vi "Test 3.vi"() -> ()   [LabVIEW 2016, in "Drona basic.lvlib"]
uses:
  Drona basic.lvlib
  Test 2.vi
panel:
  in  "Tab Control":enum32{"Page 1", "Page 2"}(tab)
  in  "Numeric 3":i32=100
  in  "Boolean":bool
  in  "Numeric 2":dbl
  in  "Numeric":dbl
  in  "error in (no error)":errorcluster
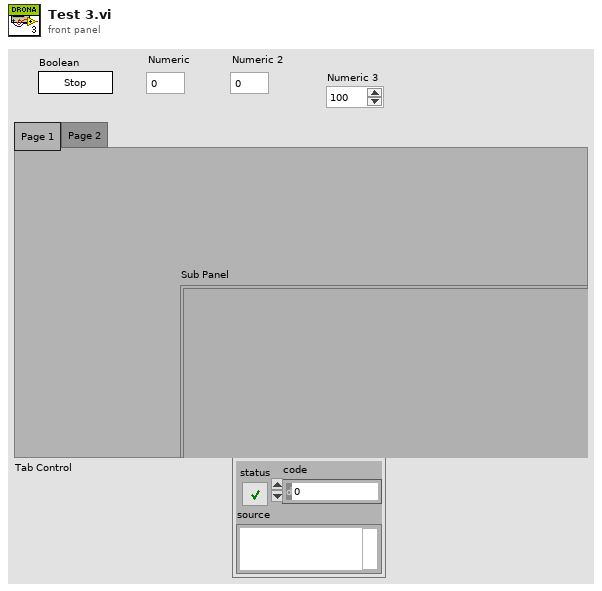
[diagram p1: front panel]
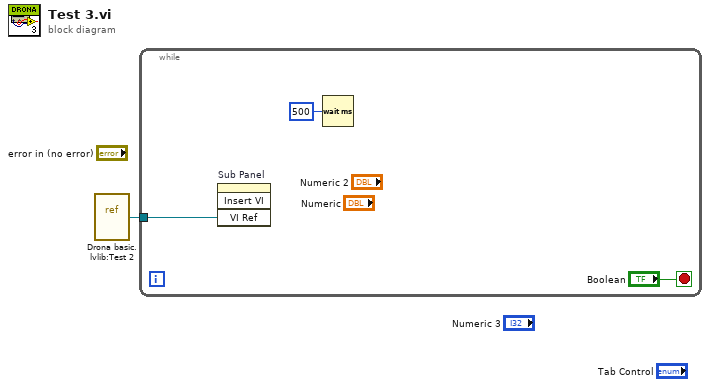
[diagram p0: block diagram]
diagram:
  n1 = vi-ref "Drona basic.lvlib:Test 2.vi"() -> (w1:refnum<vi>)
  n2 = while {
    tunnel: w1 -> [w4]
    stop <- "Boolean" stop-if-true
    n3 = invoke on="Sub Panel" class="SubPnl" method="Insert VI"("VI Ref"=w4) -> ()  [unwired: 3 in, 4 out]
    n4 = Wait (ms)(milliseconds to wait=u32 500) -> ()  [unwired: 1 out]
  }
